vi "MusicFree.vi"(8 "error in (no error)":errorcluster) -> (0 "error out":errorcluster)   [LabVIEW 2015, in "LabBASSMOD2.lvlib"]
uses:
  LabBassMOD2.lvlib
  DLL/BASSMOD.dll
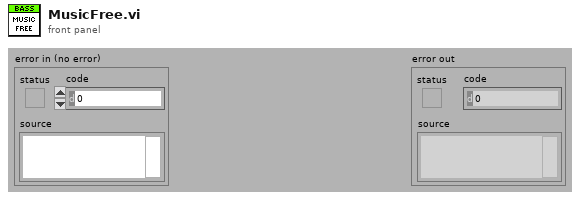
[diagram p1: front panel]
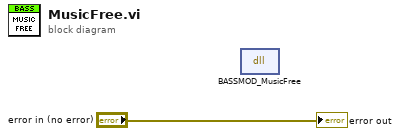
[diagram p0: block diagram]
diagram:
  n1 = dll-call lib="C:/dev/PGS/LabBASSMOD2/DLL/BASSMOD.dll" fn="BASSMOD_MusicFree"() -> ()  [unwired: 4 in, 2 out]
  "error out" <- "error in (no error)"
